vi "main(Test DQMH modules).bak.vi"() -> ()   [LabVIEW 2018, in "Application.lvlib"] (continued)
      tunnel: [w267 w1310 w1323 w1333 w1352 w1413 w1449 w1497 w1541 w1553 w1565 w1574 w1599 w1634 w1651 w1723 w1738 w1761 w1784 w1808 w1842 w1861 w1880 w1899 w1931 w1962 w1987 w2016 w2052 w2072 w2095 w2129 w2146 w2172 w2204 w2242 w2279 w2329 w2366 w2413 w2468 w2541 w2611 w2682 w2753 w2824 w2895 w2966 w3038 w3111 w3188 w3234 w3275 w3316 w3357 w3398 w3439 w3480 w3521 w3562 w3603 w3644 w3685 w3726 w3767 w3808 w3849 w3890 w3931 w3972 w4013 w4054 w4095 w4136 w4177 w4218 w4259 w4300 w4341 w4382 w4423 w4464 w4505 w4546 w4587 w4628 w4669 w4710 w4751 w4792 w4833 w4874 w4915 w4956 w4997 w5038 w5079 w5120 w5161 w5202 w5243 w5284 w5325 w5366 w5407 w5448 w5489 w5530 w5571 w5612 w5653 w5691 1 ("DUT channel (1-11)") 1 ("DUT channel (1-11)") 1 ("DUT channel (1-11)") 1 ("DUT channel (1-11)") 1 ("DUT channel (1-11)") 1 ("DUT channel (1-11)") 2 ("DUT channel (1-11)") 2 ("DUT channel (1-11)") 2 ("DUT channel (1-11)") 2 ("DUT channel (1-11)") 2 ("DUT channel (1-11)") 2 ("DUT channel (1-11)") 3 ("DUT channel (1-11)") 3 ("DUT channel (1-11)") 3 ("DUT channel (1-11)") 3 ("DUT channel (1-11)") 3 ("DUT channel (1-11)") 3 ("DUT channel (1-11)") 4 ("DUT channel (1-11)") 4 ("DUT channel (1-11)") 4 ("DUT channel (1-11)") 4 ("DUT channel (1-11)") 4 ("DUT channel (1-11)") 4 ("DUT channel (1-11)") 5 ("DUT channel (1-11)") 5 ("DUT channel (1-11)") 5 ("DUT channel (1-11)") 5 ("DUT channel (1-11)") 5 ("DUT channel (1-11)") 5 ("DUT channel (1-11)") 6 ("DUT channel (1-11)") 6 ("DUT channel (1-11)") 6 ("DUT channel (1-11)") 6 ("DUT channel (1-11)") 6 ("DUT channel (1-11)") 6 ("DUT channel (1-11)") 7 ("DUT channel (1-11)") 7 ("DUT channel (1-11)") 7 ("DUT channel (1-11)") 7 ("DUT channel (1-11)") 7 ("DUT channel (1-11)") 7 ("DUT channel (1-11)") 8 ("DUT channel (1-11)") 8 ("DUT channel (1-11)") 8 ("DUT channel (1-11)") 8 ("DUT channel (1-11)") 8 ("DUT channel (1-11)") 8 ("DUT channel (1-11)") 9 ("DUT channel (1-11)") 9 ("DUT channel (1-11)") 9 ("DUT channel (1-11)") 9 ("DUT channel (1-11)") 9 ("DUT channel (1-11)") 9 ("DUT channel (1-11)") 10 ("DUT channel (1-11)") 10 ("DUT channel (1-11)") 10 ("DUT channel (1-11)") 10 ("DUT channel (1-11)") 10 ("DUT channel (1-11)") 10 ("DUT channel (1-11)")] -> w236
      tunnel: w235 -> [w268 w1310 w1323 w1333 w1352 w1413 w1449 w1497 w1541 w1553 w1565 w1574 w1599 w1634 w1651 w1723 w1738 w1761 w1784 w1808 w1842 w1861 w1880 w1899 w1931 w1962 w1987 w2016 w2052 w2072 w2095 w2129 w2146 w2172 w2204 w2242 w2279 w2329 w2366 w2413 _ _ _ _ _ _ _ _ _ _ _ w3234 w3275 w3316 w3357 w3398 w3439 w3480 w3521 w3562 w3603 w3644 w3685 w3726 w3767 w3808 w3849 w3890 w3931 w3972 w4013 w4054 w4095 w4136 w4177 w4218 w4259 w4300 w4341 w4382 w4423 w4464 w4505 w4546 w4587 w4628 w4669 w4710 w4751 w4792 w4833 w4874 w4915 w4956 w4997 w5038 w5079 w5120 w5161 w5202 w5243 w5284 w5325 w5366 w5407 w5448 w5489 w5530 w5571 w5612 w5653 w5691 _ _ _ _ _ _ _ _ _ _ _ _ _ _ _ _ _ _ _ _ _ _ _ _ _ _ _ _ _ _ _ _ _ _ _ _ _ _ _ _ _ _ _ _ _ _ _ _ _ _ _ _ _ _ _ _ _ _ _ _]
      tunnel: [w265 w1309 w1322 w1332 w1354 w1401 w1448 w1496 w1540 w1552 w1564 w1573 w1598 w1633 w1650 w1722 w1737 w1760 w1783 w1807 w1841 w1860 w1879 w1898 w1930 w1961 w1986 w2015 w2051 w2071 w2094 w2128 w2145 w2171 w2207 w2241 w2278 w2328 w2357 w2412 w2446 w2540 w2610 w2681 w2752 w2823 w2894 w2965 w3037 w3110 w3187 w3229 w3271 w3312 w3353 w3394 w3438 w3476 w3517 w3558 w3599 w3640 w3681 w3722 w3763 w3804 w3845 w3885 w3929 w3968 w4009 w4050 w4091 w4132 w4173 w4214 w4255 w4296 w4337 w4378 w4418 w4460 w4501 w4542 w4583 w4624 w4665 w4706 w4747 w4787 w4829 w4870 w4911 w4952 w4993 w5033 w5075 w5115 w5157 w5197 w5238 w5280 w5321 w5361 w5403 w5444 w5485 w5526 w5567 w5608 w5649 w5690 w5698 w5755 w5812 w5868 w5926 w5982 w6039 w6096 w6153 w6210 w6267 w6324 w6382 w6439 w6496 w6553 w6610 w6667 w6724 w6781 w6837 w6895 w6951 w7008 w7066 w7122 w7180 w7236 w7294 w7350 w7407 w7464 w7522 w7579 w7635 w7692 w7749 w7806 w7863 w7920 w7977 w8034 w8091 w8151 w8205 w8263 w8319 w8377 w8434 w8491 w8547 w8604 w8661 w8718 w8775 w8832 w8893 w8952 w9011 w9070] -> w234
      tunnel: w233 -> [w266 w1309 w1322 w1332 w1354 w1401 w1448 w1496 w1540 w1552 w1564 w1573 w1598 w1633 w1650 w1722 w1737 w1760 w1783 w1807 w1841 w1860 w1879 w1898 w1930 w1961 w1986 w2015 w2051 w2071 w2094 w2128 w2145 w2171 w2207 w2241 w2278 w2328 w2357 w2412 w2446 w2540 w2610 w2681 w2752 w2823 w2894 w2965 w3037 w3110 w3187 _ _ _ _ _ _ _ _ _ _ _ _ _ _ _ _ _ _ _ _ _ _ _ _ _ _ _ _ _ _ _ _ _ _ _ _ _ _ _ _ _ _ _ _ _ _ _ _ _ _ _ _ _ _ _ _ _ _ _ _ w5690 _ _ _ _ _ _ _ _ _ _ _ _ _ _ _ _ _ _ _ _ _ _ _ _ _ _ _ _ _ _ _ _ _ _ _ _ _ _ _ _ _ _ _ _ _ _ _ _ _ _ _ _ _ _ _ _ _ _ _ _]
      tunnel: w230 -> [w273 _ _ _ _ _ _ _ _ _ _ _ _ _ _ _ _ _ _ _ _ _ _ _ _ _ _ _ w2043 _ _ _ _ _ _ _ _ _ _ _ _ _ _ _ _ _ _ _ _ _ _ _ _ _ _ _ _ _ _ _ _ _ _ _ _ _ _ _ _ _ _ _ _ _ _ _ _ _ _ _ _ _ _ _ _ _ _ _ _ _ _ _ _ _ _ _ _ _ _ _ _ _ _ _ _ _ _ _ _ _ _ _ _ _ _ _ _ _ _ _ _ _ _ _ _ _ _ _ _ _ _ _ _ _ _ _ _ _ _ _ _ _ _ _ _ _ _ _ _ _ _ _ _ _ _ _ _ _ _ _ _ _ _ _ _ _ _ _ _ _ _ _]
      tunnel: [_ _ _ _ _ _ _ _ _ _ _ _ _ _ _ _ _ _ _ _ _ _ _ _ _ _ _ _ _ _ _ _ _ _ _ _ _ _ TRUE _ _ _ _ _ _ _ _ _ _ _ _ _ _ _ _ _ _ _ _ _ _ _ _ _ _ _ _ _ _ _ _ _ _ _ _ _ _ _ _ _ _ _ _ _ _ _ _ _ _ _ _ _ _ _ _ _ _ _ _ _ _ _ _ _ _ _ _ _ _ _ _ _ _ _ _ _ _ _ _ _ _ _ _ _ _ _ _ _ _ _ _ _ _ _ _ _ _ _ _ _ _ _ _ _ _ _ _ _ _ _ _ _ _ _ _ _ _ _ _ _ _ _ _ _ _ _ _ _ _ _ _ _] -> w229
      tunnel: [w269 w1308 w1316 w1328 w1350 w1411 "Test Completed!!!!" w1488 w1539 w1551 w1563 w1571 w1594 w1632 "Initialize Apps" w1700 w1733 w1756 w1779 w1802 w1836 w1855 w1874 w1893 w1919 w1956 w1983 w2012 w2038 "HV-60D ready!!!!!!!!!!!!!!!!" w2088 w2125 w2140 w2164 w2201 w2236 w2271 w2321 w2359 "Shorted Circuit Test" "Test Channel 1" "Test Channel 2" "Test Channel 3" "Test Channel 4" "Test Channel 5" "Test Channel 6" "Test Channel 7" "Test Channel 8" "Test Channel 9" "Test Channel 10" "Test Channel 10" w3232 w3274 w3315 w3356 w3397 w3436 w3479 w3520 w3561 w3602 w3643 w3684 w3725 w3766 w3807 w3848 w3889 w3928 w3971 w4012 w4053 w4094 w4135 w4176 w4217 w4258 w4299 w4340 w4381 w4422 w4463 w4504 w4545 w4586 w4627 w4668 w4709 w4750 w4791 w4832 w4873 w4914 w4955 w4996 w5037 w5078 w5119 w5160 w5201 w5242 w5283 w5324 w5365 w5406 w5447 w5488 w5529 w5570 w5611 w5652 w5689 w5707 w5764 w5821 w5878 w5935 w5992 w6049 w6106 w6163 w6220 w6277 w6334 w6391 w6448 w6506 w6563 w6620 w6677 w6734 w6791 w6848 w6905 w6962 w7019 w7076 w7133 w7190 w7247 w7304 w7361 w7418 w7475 w7532 w7589 w7646 w7703 w7760 w7818 w7874 w7931 w7988 w8045 w8102 w8159 w8216 w8273 w8332 w8387 w8444 w8501 w8558 w8615 w8673 w8729 w8786 w8843 w8903 w8962 w9021 w9080] -> w226
      tunnel: w225 -> [w270 w1308 w1316 w1328 w1350 w1411 _ _ w1539 w1551 w1563 w1571 w1594 w1632 _ w1700 w1733 w1756 w1779 w1802 w1836 w1855 w1874 w1893 w1919 w1956 w1983 w2012 w2038 _ w2088 w2125 w2140 w2164 w2201 w2236 w2271 w2321 w2359 _ _ _ _ _ _ _ _ _ _ _ _ w3231 w3273 w3314 w3355 w3396 w3435 w3478 w3519 w3560 w3601 w3642 w3683 w3724 w3765 w3806 w3847 w3888 w3927 w3970 w4011 w4052 w4093 w4134 w4175 w4216 w4257 w4298 w4339 w4380 w4421 w4462 w4503 w4544 w4585 w4626 w4667 w4708 w4749 w4790 w4831 w4872 w4913 w4954 w4995 w5036 w5077 w5118 w5159 w5200 w5241 w5282 w5323 w5364 w5405 w5446 w5487 w5528 w5569 w5610 w5651 w5689 _ _ _ _ _ _ _ _ _ _ _ _ _ _ _ _ _ _ _ _ _ _ _ _ _ _ _ _ _ _ _ _ _ _ _ _ _ _ _ _ _ _ _ _ _ _ _ _ _ _ _ _ _ _ _ _ _ _ _ _]
      tunnel: w223 -> [_ _ _ _ _ _ w1427 _ _ _ _ _ _ _ _ _ _ _ _ _ _ _ _ _ _ _ _ _ _ _ _ _ _ _ _ _ _ _ _ _ _ _ _ _ _ _ _ _ _ _ _ _ _ _ _ _ _ _ _ _ _ _ _ _ _ _ _ _ _ _ _ _ _ _ _ _ _ _ _ _ _ _ _ _ _ _ _ _ _ _ _ _ _ _ _ _ _ _ _ _ _ _ _ _ _ _ _ _ _ _ _ _ _ _ _ _ _ _ _ _ _ _ _ _ _ _ _ _ _ _ _ _ _ _ _ _ _ _ _ _ _ _ _ _ _ _ _ _ _ _ _ _ _ _ _ _ _ _ _ _ _ _ _ _ _ _ _ _ _ _ _ _]
      frame "Apps.WaitForEvent", Default {
        n141 = event shown="[26] <CE14_v2 Broadcast Events.CE14 response data>: User Event" {
          selector: w282 -> [_ w310 _ _ _ _ _ _ _ _ _ _ _ _ _ _ _ _ _ _ _ _ _ _ _ _ _ _ _ _ _ _ _ _ _ _ _ _ _ _ _ _]
          dyn-events: [_ w310 _ _ _ _ _ _ _ _ _ _ _ _ _ _ _ _ _ _ _ _ _ _ _ _ _ _ _ _ _ _ _ _ _ _ _ _ _ _ _ _] -> w281
          timeout: w271 -> [_ _ _ _ _ _ _ _ _ _ _ _ _ _ _ _ _ _ _ _ _ _ _ _ _ _ _ _ _ _ _ _ _ _ _ _ _ _ _ _ _ _]
          tunnel: [w289 w305 w323 w346 w361 w379 w394 w479 w491 w502 w510 w532 w551 w568 w580 w601 w623 w658 w677 w694 w718 w737 w756 w785 w825 w845 w873 w981 w1012 w1035 w1056 w1077 w1098 w1119 w1140 w1161 w1182 w1203 w1224 w1240 w1265 w1290] -> w283
          tunnel: w271 -> [w289 w305 w324 w346 w361 w379 w393 w479 w491 w502 w510 w532 w551 w568 w580 w601 w623 w658 w677 w694 w718 w737 w756 w785 w825 w845 w873 w981 w1012 w1035 w1056 w1077 w1098 w1119 w1140 w1161 w1182 w1203 w1224 w1240 w1265 w1290]
          tunnel: [w293 w309 _ w337 _ w376 w384 w473 w483 w497 w508 w527 w546 w560 w576 w599 w621 w651 w672 w691 w716 w735 w754 w779 w817 w839 w869 w980 w1009 w1033 w1054 w1075 w1096 w1117 w1138 w1159 w1180 w1201 w1222 w1238 w1262 w1287] -> w279
          tunnel: w278 -> [w287 w309 _ w339 _ w378 w398 w474 w485 w501 w507 w526 w545 w561 w575 w598 w620 w650 w671 w690 w715 w734 w753 w778 w819 w843 w868 w979 w1010 w1034 w1055 w1076 w1097 w1118 w1139 w1160 w1181 w1202 w1223 w1237 w1261 w1288]
          tunnel: w277 -> [w290 w303 w325 w341 _ w367 w400 w477 w487 w500 w513 w531 w550 _ w570 w606 w627 w655 w676 w702 w721 w740 w761 w782 w824 w846 w870 w969 w1006 w1030 w1051 w1072 w1093 w1114 w1135 w1157 w1177 w1198 w1219 w1231 w1256 w1281]
          tunnel: [w294 w312 w330 w345 w360 w375 w399 w478 w489 w495 w509 w529 w547 w567 w577 w600 w622 w652 w673 w693 w717 w736 w755 w784 w820 w840 w871 w982 w1005 w1028 w1049 w1070 w1091 w1112 w1133 w1155 w1175 w1196 w1217 w1239 w1264 w1289] -> w276
          tunnel: w275 -> [w294 w312 w330 w345 w360 w375 w399 w478 w489 w495 w509 w529 w547 w567 w577 w600 w622 w652 w673 w693 w717 w736 w755 w784 w820 _ w872 w982 w1005 w1028 w1049 w1070 w1091 w1112 w1133 w1155 w1175 w1196 w1217 w1239 w1264 w1289]
          tunnel: w274 -> [_ _ _ w335 _ _ w386 _ _ _ _ _ _ _ _ _ _ _ _ _ _ _ _ _ _ _ _ _ _ w1027 w1046 w1066 w1087 w1108 w1129 w1150 w1171 w1192 w1213 _ _ _]
          tunnel: w272 -> [w292 w311 _ _ _ _ _ _ _ _ w506 w525 w544 _ w574 w597 w619 w649 w670 w689 w714 w733 w752 w777 w816 w841 w866 w978 _ _ _ _ _ _ _ _ _ _ _ w1236 w1263 w1286]
          tunnel: w273 -> [_ _ _ _ _ _ _ _ _ _ _ _ _ _ _ _ _ _ _ _ _ _ _ _ _ _ _ _ _ _ _ _ _ _ _ _ _ _ _ _ _ _]
          tunnel: w268 -> [w285 w307 w328 w343 w358 w373 w388 w471 w481 w493 w504 w523 w542 w565 w572 w595 _ w647 w668 w687 w712 w731 w750 w774 w814 w835 w863 w965 w1003 _ _ _ _ _ _ _ _ _ _ w1234 w1259 w1284]
          tunnel: w270 -> [w286 _ w329 w344 w359 w374 _ _ w482 w494 w505 w524 w543 w566 w573 w596 w618 w648 w669 w688 w713 w732 w751 w776 w815 w836 w864 w966 w1004 w1023 w1044 w1065 w1086 w1107 w1128 w1149 w1170 w1191 w1212 w1235 w1260 w1285]
          tunnel: [w286 "Wait for JIG lock" w329 w344 w359 w374 "Start Auto Test" "Settings" w482 w494 w505 w524 w543 w566 w573 w596 w618 w648 w669 w688 w713 w732 w751 w776 w815 w836 w864 w966 w1004 w1023 w1044 w1065 w1086 w1107 w1128 w1149 w1170 w1191 w1212 w1235 w1260 w1285] -> w269
          tunnel: [w285 w307 w328 w343 w358 w373 w388 w471 w481 w493 w504 w523 w542 w565 w572 w595 w615 w647 w668 w687 w712 w731 w750 w774 w814 w835 w862 w965 w1003 1 ("DUT channel (1-11)") 2 ("DUT channel (1-11)") 3 ("DUT channel (1-11)") 4 ("DUT channel (1-11)") 5 ("DUT channel (1-11)") 6 ("DUT channel (1-11)") 7 ("DUT channel (1-11)") 8 ("DUT channel (1-11)") 9 ("DUT channel (1-11)") 10 ("DUT channel (1-11)") w1234 w1259 w1284] -> w267
          tunnel: w266 -> [w284 w306 w327 w342 w357 w372 w387 w470 w480 w492 w503 w522 w541 w564 w571 w594 w617 w646 w667 w686 w711 w730 w749 _ w813 w834 w858 w964 w1002 w1021 w1042 w1063 w1084 w1105 w1126 w1147 w1168 w1189 w1210 w1230 w1255 w1280]
          tunnel: [w284 w306 w327 w342 w357 w372 w387 w470 w480 w492 w503 w522 w541 w564 w571 w594 w617 w646 w667 w686 w711 w730 w749 w770 w813 w834 w857 w964 w1002 w1021 w1042 w1063 w1084 w1105 w1126 w1147 w1168 w1189 w1210 w1230 w1255 w1280] -> w265
          tunnel: w264 -> [_ _ _ _ _ _ _ _ _ _ _ _ _ _ _ _ _ _ _ _ _ _ _ _ _ _ w861 _ _ _ _ _ _ _ _ _ _ _ _ _ _ _]
          event Timeout {
            n142 = event-data() -> ()  [unwired: 1 in, 1 out]
            n143 = disable-structure shown="LOGGING==TRUE" {
              disable-tunnel: w292 -> [w295 _]
              frame condition #0 (active) {
                n144 = Empty String/Path?(string/path=w295) -> (empty?=w302:bool)
                n145 = Select(t="Quece timeout", s=w302, f=w295) -> (s? t:f=w300:string)
                n146 = Format Into String(format string=": %s", initial string=w300, "UI timeout") -> (resulting string=w297:string)  [unwired: 1 in, 1 out]
                n147 = call "string log (SubVI).vi"("Enum"=enum16{"Init", "Log", "Read"}."Log", "state Name"=w297) -> ()  [unwired: 8 in, 2 out]
              }
              frame condition #1 {
              }
            }
            n148 = call "App enquece.vi"("command"="Apps.WaitingForTrigger", "queue in"=w290) -> ("error out"=w288:errorcluster)  [unwired: 8 in, 1 out]
            n149 = Merge Errors(w287, w288) -> (w293:errorcluster)
          }
          event "Test": Value Change {
            n150 = event-data() -> ()  [unwired: 1 in, 2 out]
            n151 = disable-structure shown="Default" {
              disable-tunnel: w311 -> [w315 _]
              frame condition #0 (active) {
                n152 = Empty String/Path?(string/path=w315) -> (empty?=w322:bool)
                n153 = Select(t="Quece timeout", s=w322, f=w315) -> (s? t:f=w320:string)
                n154 = Format Into String(format string=": %s", initial string=w320, "Test") -> (resulting string=w317:string)  [unwired: 1 in, 1 out]
                n155 = call "string log (SubVI).vi"("Enum"=enum16{"Init", "Log", "Read"}."Log", "state Name"=w317) -> ()  [unwired: 8 in, 2 out]
              }
              frame condition #1 {
              }
            }
            n156 = call "App enquece.vi"("command"="Apps.AutoMode", "queue in"=w303) -> ()  [unwired: 8 in, 2 out]
            n157 = disable-structure shown="Disabled" {
              frame Disabled {
                n158 = Select(t=100, f=-1) -> ()  [unwired: 1 in, 1 out]
              }
              frame Enabled {
              }
            }
          }
          event "Auto/Man": Value Change {
            n159 = event-data() -> ("NewVal"=w326:bool)  [unwired: 1 in, 5 out]
            n160 = case shown="True" w326 {
              tunnel: w325 -> [_ w333]
              tunnel: [-1 w332] -> w323
              tunnel: w324 -> [_ w332]
              frame False {
              }
              frame True {
                n161 = call "App enquece.vi"("command"="Apps.AutoMode", "queue in"=w333) -> ()  [unwired: 8 in, 2 out]
              }
            }
          }
          event "Test Single DRV": Value Change {
            n162 = event-data() -> ()  [unwired: 1 in, 1 out]
            n163 = case shown="1.." "DRV number" {
              selector: "DRV number" -> [_ w349]
              tunnel: ["MEAS.AllRelaysOFF" w352] -> w340
              tunnel: w335 -> [w347 _]
              frame 0, Default {
                n164 = call "reset DRV UI (SubVI).vi"("Ref  in"=w347) -> ()  [unwired: 9 in, 2 out]
              }
              frame 1.. {
                n165 = Format Into String(format string="%d%s", initial string="Test DRV ", w349, "A" ("input 3")) -> (resulting string=w352:string)  [unwired: 1 in, 1 out]
              }
            }
            n166 = call "App enquece.vi"("command"=w340, "queue in"=w341) -> ("error out"=w338:errorcluster)  [unwired: 8 in, 1 out]
            n167 = Merge Errors(w339, w338) -> (w337:errorcluster)
          }
          event "DMM query": Value Change {
            n168 = event-data() -> ()  [unwired: 1 in, 6 out]
            n169 = flat-sequence {
              tunnel: [w364] -> w355
              frame #0 {
                w362 = ""
                n170 = Wait (ms)(milliseconds to wait=u32 100) -> ()  [unwired: 1 out]
                n171 = local write "DMM func?"(w362) -> ()
                n172 = local write "DMM range?"(w362) -> ()
                n173 = xnode "Error Ring"() -> ("error out"=w364:errorcluster)
              }
            }
            n174 = call "Query func.vi"("error in"=w355) -> ("String"=→"DMM func?":string)  [unwired: 8 in, 2 out]
            n175 = call "query range.vi"("error in"=w355) -> ("String"=→"DMM range?":string)  [unwired: 8 in, 2 out]
          }
          event "VIEW": Value Change {
            n176 = event-data() -> ()  [unwired: 1 in, 1 out]
            n177 = disable-structure shown="Disabled" {
              frame Disabled {
                n178 = Initialize Array(FALSE, 6 ("dimension size"), 10 ("dimension size")) -> (w380:bool[][])
                n179 = local write "Short DRV"(w380) -> ()
              }
              frame Enabled {
              }
            }
            n180 = call "App enquece.vi"("command"="Apps.UI Update 1", "queue in"=w367) -> ()  [unwired: 8 in, 2 out]
            n181 = invoke class="VI" method="FP.Open"("State"=T18."Hidden") -> (error out=w371:errorcluster)  [unwired: 4 in, 4 out]
            n182 = call "View DRV data.vi"("error in (no error)"=w371) -> ("error out"=w370:errorcluster)  [unwired: 10 in]
            n183 = invoke class="VI" method="FP.Open"(error in=w370, "State"=T18."Standard") -> (error out=w377:errorcluster)  [unwired: 3 in, 4 out]
            n184 = Merge Errors(w378, w377) -> (w376:errorcluster)
          }
          event User Event {
            # "#HungNotes:\nStart HV60D from this frame (check new board  installed)"
            # "Stop Timeout event"
            n185 = event-data() -> ("new board?"=w392:bool, "new trigger"=→"new Trigger?":bool, "last trigger"=→"last Trigger?":bool)  [unwired: 1 in, 1 out]
            "New board?" <- w392
            n186 = call "reset DRV UI (SubVI).vi"("Ref  in"=w386) -> ()  [unwired: 9 in, 2 out]
            n187 = case shown="True" w392 {
              tunnel: w400 -> [_ w402]
              tunnel: [_ w401] -> w385
              frame False {
              }
              frame True {
                n188 = case shown="\"Pinpoint_JIG\"" "Enum" {
                  tunnel: [w416 w433 w444 w463] -> w403
                  frame "All DRV" {
                    n189 = Build Array("Test Shorted Circuits", "Timer Start", "Test Channel 1", "Test Channel 2", "Test Channel 3", "Test Channel 4", "Test Channel 5", "Test Channel 6") -> (w408:string[])
                    n190 = Build Array("Test Channel 7", "Test Channel 8", "Test Channel 9", "Test Channel 10", "Timer Stop") -> (w417:string[])
                    n191 = Build Array("MEAS.AllRelaysOFF", "MEAS.Reset JIG", "Apps.UI Update 2") -> (w409:string[])
                    n192 = Build Array (concatenate)(w408, w417, w409) -> (w416:string[])
                  }
                  frame "Fixxed" {
                    n193 = Build Array("Test Shorted Circuits", "Timer Start", "Test Channel 1", "Test Channel 2", "Test Channel 3", "Test Channel 4", "Test Channel 5", "Test Channel 6", "Test Channel 7") -> (w435:string[])
                    n194 = Build Array("MEAS.AllRelaysOFF", "MEAS.Reset JIG", "Apps.UI Update 2") -> (w429:string[])
                    n195 = Build Array (concatenate)(w435, "Timer Stop", w429) -> (w433:string[])
                  }
                  frame "Pinpoint_JIG" {
                    n196 = Build Array("Test Channel 8", "Test Channel 9", "Test Channel 10") -> (w448:string[])
                    n197 = Build Array("Test Shorted Circuits", "Timer Start") -> (w445:string[])
                    n198 = Build Array("MEAS.AllRelaysOFF", "MEAS.Reset JIG", "Apps.UI Update 2") -> (w447:string[])
                    n199 = Build Array (concatenate)(w445, w448, "Timer Stop", w447) -> (w444:string[])
                  }
                  frame "00037845(M26)" {
                    n200 = Build Array("Test Channel 8", "Test Channel 9", "Test Channel 10A", "Timer Stop") -> (w458:string[])
                    n201 = Build Array("Test Shorted Circuits", "Timer Start") -> (w464:string[])
                    n202 = Build Array("MEAS.AllRelaysOFF", "MEAS.Reset JIG", "Apps.UI Update 2") -> (w457:string[])
                    n203 = Build Array (concatenate)(w464, w458, w457) -> (w463:string[])
                  }
                }
                n204 = for {
                  tunnel: [w407] -> w401 mode=indexing
                  tunnel: w403 -> [w406] mode=indexing
                  tunnel: w402 -> [w405]
                  n205 = call "App enquece.vi"("command"=w406, "queue in"=w405) -> ("error out"=w407:errorcluster)  [unwired: 8 in, 1 out]
                }
              }
            }
            n206 = control-ref of="DRV 61"() -> (w390:refnum<vi>)
            n207 = property class="ColBox"(reference=w390, "Value"=u32 10000536 ("DRV 1")) -> ()  [unwired: 1 in, 2 out]
            n208 = Select(t=-1, s=w392, f=w393) -> (s? t:f=w394:i32)
            n209 = Merge Errors(w398, w385) -> (w384:errorcluster)
          }
          event "Settings": Value Change {
            n210 = event-data() -> ()  [unwired: 1 in, 6 out]
            n211 = call "App enquece.vi"("command"="INIT.Read DRV code", "queue in"=w477) -> ("error out"=w475:errorcluster)  [unwired: 8 in, 1 out]
            n212 = Merge Errors(w474, w475) -> (w473:errorcluster)
          }
          event Panel Close? {
            n213 = event-data() -> ()  [unwired: 1 in, 4 out]
            n214 = call "App enquece.vi"("Priority Enquece"=TRUE, "command"="Apps.Exit", "queue in"=w487) -> ("error out"=w484:errorcluster)  [unwired: 7 in, 1 out]
            n215 = Merge Errors(w485, w484) -> (w483:errorcluster)
            n216 = event-data("Discard?"=TRUE) -> ()  [unwired: 1 in, 1 out]
          }
          event "Exit": Value Change {
            n217 = event-data() -> ()  [unwired: 1 in, 1 out]
            n218 = call "App enquece.vi"("Priority Enquece"=TRUE, "command"="Apps.Exit", "queue in"=w500) -> ("error out"=w499:errorcluster)  [unwired: 7 in, 1 out]
            n219 = Merge Errors(w501, w499) -> (w497:errorcluster)
          }
          event "check connected": Value Change {
            n220 = event-data() -> ()  [unwired: 1 in, 1 out]
            n221 = disable-structure shown="LOGGING==TRUE" {
              disable-tunnel: w506 -> [w514 _]
              frame condition #0 (active) {
                n222 = Empty String/Path?(string/path=w514) -> (empty?=w521:bool)
                n223 = Select(t="Quece timeout", s=w521, f=w514) -> (s? t:f=w519:string)
                n224 = Format Into String(format string=": %s", initial string=w519, "Check connected") -> (resulting string=w516:string)  [unwired: 1 in, 1 out]
                n225 = call "string log (SubVI).vi"("Enum"=enum16{"Init", "Log", "Read"}."Log", "state Name"=w516) -> ()  [unwired: 8 in, 2 out]
              }
              frame condition #1 {
              }
            }
            n226 = call "App enquece.vi"("command"="MEAS.Read EMIC connected", "queue in"=w513) -> ("error out"=w511:errorcluster)  [unwired: 8 in, 1 out]
            n227 = Merge Errors(w507, w511) -> (w508:errorcluster)
          }
          event "Open COM eMIC": Value Change {
            n228 = event-data() -> ()  [unwired: 1 in, 1 out]
            n229 = disable-structure shown="LOGGING==TRUE" {
              disable-tunnel: w525 -> [w533 _]
              frame condition #0 (active) {
                n230 = Empty String/Path?(string/path=w533) -> (empty?=w540:bool)
                n231 = Select(t="Quece timeout", s=w540, f=w533) -> (s? t:f=w538:string)
                n232 = Format Into String(format string=": %s", initial string=w538, "Open COM eMIC") -> (resulting string=w535:string)  [unwired: 1 in, 1 out]
                n233 = call "string log (SubVI).vi"("Enum"=enum16{"Init", "Log", "Read"}."Log", "state Name"=w535) -> ()  [unwired: 8 in, 2 out]
              }
              frame condition #1 {
              }
            }
            n234 = call "App enquece.vi"("command"="INIT.Open COM EMIC", "queue in"=w531) -> ("error out"=w530:errorcluster)  [unwired: 8 in, 1 out]
            n235 = Merge Errors(w526, w530) -> (w527:errorcluster)
          }
          event "Read trigger": Value Change {
            n236 = event-data() -> ()  [unwired: 1 in, 1 out]
            n237 = disable-structure shown="LOGGING==TRUE" {
              disable-tunnel: w544 -> [w552 _]
              frame condition #0 (active) {
                n238 = Empty String/Path?(string/path=w552) -> (empty?=w559:bool)
                n239 = Select(t="Quece timeout", s=w559, f=w552) -> (s? t:f=w557:string)
                n240 = Format Into String(format string=": %s", initial string=w557, "Read Trigger") -> (resulting string=w554:string)  [unwired: 1 in, 1 out]
                n241 = call "string log (SubVI).vi"("Enum"=enum16{"Init", "Log", "Read"}."Log", "state Name"=w554) -> ()  [unwired: 8 in, 2 out]
              }
              frame condition #1 {
              }
            }
            n242 = call "App enquece.vi"("command"="MEAS.Read TRIGGER", "queue in"=w550) -> ("error out"=w548:errorcluster)  [unwired: 8 in, 1 out]
            n243 = Merge Errors(w545, w548) -> (w546:errorcluster)
          }
          event "Set trigger value": Value Change {
            n244 = event-data() -> ()  [unwired: 1 in, 6 out]
            n245 = call "SET trigger value.vi"("Boolean"="set value") -> ("error out"=w562:errorcluster)  [unwired: 10 in]
            n246 = Merge Errors(w561, w562) -> (w560:errorcluster)
          }
          event "Read Optos": Value Change {
            n247 = event-data() -> ()  [unwired: 1 in, 1 out]
            n248 = disable-structure shown="LOGGING==TRUE" {
              disable-tunnel: w574 -> [w586 _]
              frame condition #0 (active) {
                n249 = Empty String/Path?(string/path=w586) -> (empty?=w593:bool)
                n250 = Select(t="Quece timeout", s=w593, f=w586) -> (s? t:f=w591:string)
                n251 = Format Into String(format string=": %s", initial string=w591, "Read Optos") -> (resulting string=w588:string)  [unwired: 1 in, 1 out]
                n252 = call "string log (SubVI).vi"("Enum"=enum16{"Init", "Log", "Read"}."Log", "state Name"=w588) -> ()  [unwired: 8 in, 2 out]
              }
              frame condition #1 {
              }
            }
            n253 = flat-sequence {
              tunnel: w570 -> [w581]
              tunnel: [w581] -> w569
              frame #0 {
                n254 = Initialize Array(FALSE, 6 ("dimension size"), 10 ("dimension size")) -> (w585:bool[][])
                n255 = local write "Short DRV"(w585) -> ()
              }
            }
            n256 = call "App enquece.vi"("command"="MEAS.Read Optos", "queue in"=w569) -> ("error out"=w578:errorcluster)  [unwired: 8 in, 1 out]
            n257 = Merge Errors(w575, w578) -> (w576:errorcluster)
          }
          event "Select DMM's Current Input": Value Change {
            n258 = event-data() -> ()  [unwired: 1 in, 1 out]
            n259 = disable-structure shown="LOGGING==TRUE" {
              disable-tunnel: w597 -> [w607 _]
              frame condition #0 (active) {
                n260 = Empty String/Path?(string/path=w607) -> (empty?=w614:bool)
                n261 = Select(t="Quece timeout", s=w614, f=w607) -> (s? t:f=w612:string)
                n262 = Format Into String(format string=": %s", initial string=w612, "DMM Current Input") -> (resulting string=w609:string)  [unwired: 1 in, 1 out]
                n263 = call "string log (SubVI).vi"("Enum"=enum16{"Init", "Log", "Read"}."Log", "state Name"=w609) -> ()  [unwired: 8 in, 2 out]
              }
              frame condition #1 {
              }
            }
            n264 = To Variant(anything="mux2-1(DMM I) encode") -> (Variant=w603:variant)
            n265 = call "App enquece.vi"("command data"=w603, "command"="MEAS.Sel Input Current", "queue in"=w606) -> ("error out"=w602:errorcluster)  [unwired: 7 in, 1 out]
            n266 = Merge Errors(w598, w602) -> (w599:errorcluster)
          }
          event "DEMUX 1-10": Value Change {
            n267 = event-data() -> ()  [unwired: 1 in, 1 out]
            n268 = disable-structure shown="LOGGING==TRUE" {
              disable-tunnel: w619 -> [w638 _]
              frame condition #0 (active) {
                n269 = Empty String/Path?(string/path=w638) -> (empty?=w645:bool)
                n270 = Select(t="Quece timeout", s=w645, f=w638) -> (s? t:f=w643:string)
                n271 = Format Into String(format string=": %s", initial string=w643, "demux1-10") -> (resulting string=w640:string)  [unwired: 1 in, 1 out]
                n272 = call "string log (SubVI).vi"("Enum"=enum16{"Init", "Log", "Read"}."Log", "state Name"=w640) -> ()  [unwired: 8 in, 2 out]
              }
              frame condition #1 {
              }
            }
            n273 = To Variant(anything="demux1_10(x6)_encode") -> (Variant=w625:variant)
            n274 = case shown="\"demux1_10_channel0\", Default" "demux1_10(x6)_encode" {
              tunnel: [_ 1 ("DUT channel (1-11)") 2 ("DUT channel (1-11)") 3 ("DUT channel (1-11)") 4 ("DUT channel (1-11)") 5 ("DUT channel (1-11)") 6 ("DUT channel (1-11)") 7 ("DUT channel (1-11)") 8 ("DUT channel (1-11)") 9 ("DUT channel (1-11)") 10 ("DUT channel (1-11)")] -> w615
              frame "demux1_10_channel0", Default {
              }
              frame "demux1_10_channel1" {
              }
              frame "demux1_10_channel2" {
              }
              frame "demux1_10_channel3" {
              }
              frame "demux1_10_channel4" {
              }
              frame "demux1_10_channel5" {
              }
              frame "demux1_10_channel6" {
              }
              frame "demux1_10_channel7" {
              }
              frame "demux1_10_channel8" {
              }
              frame "demux1_10_channel9" {
              }
              frame "demux1_10_channel10" {
              }
            }
            n275 = call "App enquece.vi"("command data"=w625, "command"="MEAS.demux1-10", "queue in"=w627) -> ("error out"=w624:errorcluster)  [unwired: 7 in, 1 out]
            n276 = Merge Errors(w620, w624) -> (w621:errorcluster)
          }
          event "eMIC": Value Change {
            n277 = event-data() -> ()  [unwired: 1 in, 1 out]
            n278 = disable-structure shown="LOGGING==TRUE" {
              disable-tunnel: w649 -> [w659 _]
              frame condition #0 (active) {
                n279 = Empty String/Path?(string/path=w659) -> (empty?=w666:bool)
                n280 = Select(t="Quece timeout", s=w666, f=w659) -> (s? t:f=w664:string)
                n281 = Format Into String(format string=": %s", initial string=w664, "eMIC") -> (resulting string=w661:string)  [unwired: 1 in, 1 out]
                n282 = call "string log (SubVI).vi"("Enum"=enum16{"Init", "Log", "Read"}."Log", "state Name"=w661) -> ()  [unwired: 8 in, 2 out]
              }
              frame condition #1 {
              }
            }
            n283 = To Variant(anything="eMIC 6 values") -> (Variant=w653:variant)
            n284 = call "App enquece.vi"("command data"=w653, "command"="MEAS.eMIC", "queue in"=w655) -> ("error out"=w657:errorcluster)  [unwired: 7 in, 1 out]
            n285 = Merge Errors(w650, w657) -> (w651:errorcluster)
          }
          event "connect DMM": Value Change {
            n286 = event-data() -> ()  [unwired: 1 in, 1 out]
            n287 = disable-structure shown="LOGGING==TRUE" {
              disable-tunnel: w670 -> [w678 _]
              frame condition #0 (active) {
                n288 = Empty String/Path?(string/path=w678) -> (empty?=w685:bool)
                n289 = Select(t="Quece timeout", s=w685, f=w678) -> (s? t:f=w683:string)
                n290 = Format Into String(format string=": %s", initial string=w683, "Connect DMM") -> (resulting string=w680:string)  [unwired: 1 in, 1 out]
                n291 = call "string log (SubVI).vi"("Enum"=enum16{"Init", "Log", "Read"}."Log", "state Name"=w680) -> ()  [unwired: 8 in, 2 out]
              }
              frame condition #1 {
              }
            }
            n292 = call "App enquece.vi"("command"="INIT.Open COM DMM", "queue in"=w676) -> ("error out"=w675:errorcluster)  [unwired: 8 in, 1 out]
            n293 = Merge Errors(w671, w675) -> (w672:errorcluster)
          }
          event "config DMM": Value Change {
            n294 = event-data() -> ()  [unwired: 1 in, 1 out]
            n295 = disable-structure shown="LOGGING==TRUE" {
              disable-tunnel: w689 -> [w703 _]
              frame condition #0 (active) {
                n296 = Empty String/Path?(string/path=w703) -> (empty?=w710:bool)
                n297 = Select(t="Quece timeout", s=w710, f=w703) -> (s? t:f=w708:string)
                n298 = Format Into String(format string=": %s", initial string=w708, "config DMM") -> (resulting string=w705:string)  [unwired: 1 in, 1 out]
                n299 = call "string log (SubVI).vi"("Enum"=enum16{"Init", "Log", "Read"}."Log", "state Name"=w705) -> ()  [unwired: 8 in, 2 out]
              }
              frame condition #1 {
              }
            }
            n300 = Bundle By Name(cluster=T19 {"DMM config cluster"={"DCV range"=0.0, "DCI range"=0.0, "Detector Rate"=0}, "mux2-1(DMM I) encode"=enum."DMM I (0.5)"} ("DMM all config"), "DMM config cluster.DCV range"="DCV range", "DMM config cluster.DCI range"="DCI range", "DMM config cluster.Detector Rate"="Detector Rate") -> (w697:T19)
            n301 = To Variant(anything=w697) -> (Variant=w695:variant)
            n302 = call "App enquece.vi"("command data"=w695, "command"="MEAS.Set DMM config", "queue in"=w702) -> ("error out"=w692:errorcluster)  [unwired: 7 in, 1 out]
            n303 = Merge Errors(w690, w692) -> (w691:errorcluster)
          }
          event "DMM read dual value": Value Change {
            n304 = event-data() -> ()  [unwired: 1 in, 1 out]
            n305 = disable-structure shown="LOGGING==TRUE" {
              disable-tunnel: w714 -> [w722 _]
              frame condition #0 (active) {
                n306 = Empty String/Path?(string/path=w722) -> (empty?=w729:bool)
                n307 = Select(t="Quece timeout", s=w729, f=w722) -> (s? t:f=w727:string)
                n308 = Format Into String(format string=": %s", initial string=w727, "DMM read dual value") -> (resulting string=w724:string)  [unwired: 1 in, 1 out]
                n309 = call "string log (SubVI).vi"("Enum"=enum16{"Init", "Log", "Read"}."Log", "state Name"=w724) -> ()  [unwired: 8 in, 2 out]
              }
              frame condition #1 {
              }
            }
            n310 = call "App enquece.vi"("command"="MEAS.DMM dual read", "queue in"=w721) -> ("error out"=w719:errorcluster)  [unwired: 8 in, 1 out]
            n311 = Merge Errors(w715, w719) -> (w716:errorcluster)
          }
          event "Reset JIG": Value Change {
            n312 = event-data() -> ()  [unwired: 1 in, 1 out]
            n313 = disable-structure shown="LOGGING==TRUE" {
              disable-tunnel: w733 -> [w741 _]
              frame condition #0 (active) {
                n314 = Empty String/Path?(string/path=w741) -> (empty?=w748:bool)
                n315 = Select(t="Quece timeout", s=w748, f=w741) -> (s? t:f=w746:string)
                n316 = Format Into String(format string=": %s", initial string=w746, "reset JIG") -> (resulting string=w743:string)  [unwired: 1 in, 1 out]
                n317 = call "string log (SubVI).vi"("Enum"=enum16{"Init", "Log", "Read"}."Log", "state Name"=w743) -> ()  [unwired: 8 in, 2 out]
              }
              frame condition #1 {
              }
            }
            n318 = call "App enquece.vi"("command"="MEAS.Reset JIG", "queue in"=w740) -> ("error out"=w738:errorcluster)  [unwired: 8 in, 1 out]
            n319 = Merge Errors(w734, w738) -> (w735:errorcluster)
          }
          event "TurnON/OFF +5V": Value Change {
            n320 = event-data() -> ()  [unwired: 1 in, 1 out]
            n321 = disable-structure shown="LOGGING==TRUE" {
              disable-tunnel: w752 -> [w762 _]
              frame condition #0 (active) {
                n322 = Empty String/Path?(string/path=w762) -> (empty?=w769:bool)
                n323 = Select(t="Quece timeout", s=w769, f=w762) -> (s? t:f=w767:string)
                n324 = Format Into String(format string=": %s", initial string=w767, "ON/OFF +5V") -> (resulting string=w764:string)  [unwired: 1 in, 1 out]
                n325 = call "string log (SubVI).vi"("Enum"=enum16{"Init", "Log", "Read"}."Log", "state Name"=w764) -> ()  [unwired: 8 in, 2 out]
              }
              frame condition #1 {
              }
            }
            n326 = To Variant(anything="5V Value") -> (Variant=w758:variant)
            n327 = call "App enquece.vi"("command data"=w758, "command"="MEAS.Turn+5V", "queue in"=w761) -> ("error out"=w760:errorcluster)  [unwired: 7 in, 1 out]
            n328 = Merge Errors(w753, w760) -> (w754:errorcluster)
          }
          event "mux 6-1": Value Change {
            n329 = event-data() -> ()  [unwired: 1 in, 1 out]
            n330 = disable-structure shown="LOGGING==TRUE" {
              disable-tunnel: w777 -> [w805 _]
              frame condition #0 (active) {
                n331 = Empty String/Path?(string/path=w805) -> (empty?=w812:bool)
                n332 = Select(t="Quece timeout", s=w812, f=w805) -> (s? t:f=w810:string)
                n333 = Format Into String(format string=": %s", initial string=w810, "mux6-1") -> (resulting string=w807:string)  [unwired: 1 in, 1 out]
                n334 = call "string log (SubVI).vi"("Enum"=enum16{"Init", "Log", "Read"}."Log", "state Name"=w807) -> ()  [unwired: 8 in, 2 out]
              }
              frame condition #1 {
              }
            }
            n335 = Decrement(x=w774) -> (x-1=w773:i32)
            n336 = Multiply(x=w773, y=6) -> (x*y=w771:i32)
            n337 = case shown="\"mux6_1_channel6_3\"" "mux 6-1 data" {
              tunnel: w771 -> [_ w789 w792 w795 w798 w801 w804]
              tunnel: [0 w787 w790 w793 w796 w799 w802] -> w770
              frame "mux6-1_channel0", Default {
              }
              frame "mux6_1_channel1_3" {
                n338 = Add(x=w789, y=0) -> (x+y=w787:i32)
              }
              frame "mux6_1_channel2_3" {
                n339 = Add(x=w792, y=1) -> (x+y=w790:i32)
              }
              frame "mux6_1_channel3_3" {
                n340 = Add(x=w795, y=2) -> (x+y=w793:i32)
              }
              frame "mux6_1_channel4_3" {
                n341 = Add(x=w798, y=3) -> (x+y=w796:i32)
              }
              frame "mux6_1_channel5_3" {
                n342 = Add(x=w801, y=4) -> (x+y=w799:i32)
              }
              frame "mux6_1_channel6_3" {
                n343 = Add(x=w804, y=5) -> (x+y=w802:i32)
              }
            }
            n344 = To Variant(anything="mux 6-1 data") -> (Variant=w781:variant)
            n345 = call "App enquece.vi"("command data"=w781, "command"="MEAS.mux6_1", "queue in"=w782) -> ("error out"=w780:errorcluster)  [unwired: 7 in, 1 out]
            n346 = Merge Errors(w778, w780) -> (w779:errorcluster)
          }
          event "Mux 10-1": Value Change {
            n347 = event-data() -> ()  [unwired: 1 in, 1 out]
            n348 = disable-structure shown="LOGGING==TRUE" {
              disable-tunnel: w816 -> [w826 _]
              frame condition #0 (active) {
                n349 = Empty String/Path?(string/path=w826) -> (empty?=w833:bool)
                n350 = Select(t="Quece timeout", s=w833, f=w826) -> (s? t:f=w831:string)
                n351 = Format Into String(format string=": %s", initial string=w831, "mux10-1") -> (resulting string=w828:string)  [unwired: 1 in, 1 out]
                n352 = call "string log (SubVI).vi"("Enum"=enum16{"Init", "Log", "Read"}."Log", "state Name"=w828) -> ()  [unwired: 8 in, 2 out]
              }
              frame condition #1 {
              }
            }
            n353 = To Variant(anything="mux 10-1 data") -> (Variant=w821:variant)
            n354 = call "App enquece.vi"("command data"=w821, "command"="MEAS.mux10-1", "queue in"=w824) -> ("error out"=w818:errorcluster)  [unwired: 7 in, 1 out]
            n355 = Merge Errors(w819, w818) -> (w817:errorcluster)
          }
          event "request AC-all": Value Change {
            w840 = T8 {"eMIC 1"={"ACV"=0.0, "ACI"=0.0, "pF"=0.0, "kW"=0.0, "Freq"=0.0, "kvar"=0.0}, "eMIC 2"={"ACV"=0.0, "ACI"=0.0, "pF"=0.0, "kW"=0.0, "Freq"=0.0, "kvar"=0.0}, "eMIC 3"={"ACV"=0.0, "ACI"=0.0, "pF"=0.0, "kW"=0.0, "Freq"=0.0, "kvar"=0.0}, "eMIC 4"={"ACV"=0.0, "ACI"=0.0, "pF"=0.0, "kW"=0.0, "Freq"=0.0, "kvar"=0.0}, "eMIC 5"={"ACV"=0.0, "ACI"=0.0, "pF"=0.0, "kW"=0.0, "Freq"=0.0, "kvar"=0.0}, "eMIC 6"={"ACV"=0.0, "ACI"=0.0, "pF"=0.0, "kW"=0.0, "Freq"=0.0, "kvar"=0.0}}  # eMICs cluster
            n356 = event-data() -> ()  [unwired: 1 in, 1 out]
            n357 = disable-structure shown="LOGGING==TRUE" {
              disable-tunnel: w841 -> [w847 _]
              frame condition #0 (active) {
                n358 = Empty String/Path?(string/path=w847) -> (empty?=w854:bool)
                n359 = Select(t="Quece timeout", s=w854, f=w847) -> (s? t:f=w852:string)
                n360 = Format Into String(format string=": %s", initial string=w852, "request AC") -> (resulting string=w849:string)  [unwired: 1 in, 1 out]
                n361 = call "string log (SubVI).vi"("Enum"=enum16{"Init", "Log", "Read"}."Log", "state Name"=w849) -> ()  [unwired: 8 in, 2 out]
              }
              frame condition #1 {
              }
            }
            n362 = call "FGV wait for 6 eMICs.vi"("Enum"=enum16{"Init", "count"}."Init") -> ("error out"=w837:errorcluster)  [unwired: 8 in, 2 out]
            n363 = call "App enquece.vi"("error in (no error)"=w837, "command"="MEAS.requestAC", "queue in"=w846) -> ("error out"=w842:errorcluster)  [unwired: 7 in, 1 out]
            n364 = Merge Errors(w843, w842) -> (w839:errorcluster)
          }
          event User Event {
            n365 = event-data() -> ("Module ID"=w865:i32, "Array"=w880:T24[])  [unwired: 1 in]
            n366 = Variant To Data(type=0, Variant=w861) -> (data=w859:i32)  [unwired: 1 in, 1 out]
            n367 = for {
              tunnel: w880 -> [w943] mode=indexing
              shift-right: [w939] -> w856
              shift-left: T7 {"ACV"=0.0, "ACI"=0.0, "pF"=0.0, "kW"=0.0, "Freq"=0.0, "kvar"=0.0} ("eMIC response") -> [w941]
              n368 = Unbundle By Name(w943) -> ("float"=w940:dbl, "Name"=w942:string)
              n369 = case shown="\"kVar\"" w942 {
                tunnel: w941 -> [w944 w947 w950 w953 w956 w959 w962]
                tunnel: w940 -> [_ w945 w948 w951 w955 w957 w961]
                tunnel: [w944 w946 w949 w952 w954 w958 w960] -> w939
                frame "False", Default {
                }
                frame "ACI" {
                  n370 = Bundle By Name(cluster=w947, "ACI"=w945) -> (w946:T7)
                }
                frame "kW" {
                  n371 = Bundle By Name(cluster=w950, "kW"=w948) -> (w949:T7)
                }
                frame "PF" {
                  n372 = Bundle By Name(cluster=w953, "pF"=w951) -> (w952:T7)
                }
                frame "ACV" {
                  n373 = Bundle By Name(cluster=w956, "ACV"=w955) -> (w954:T7)
                }
                frame "Freq" {
                  n374 = Bundle By Name(cluster=w959, "Freq"=w957) -> (w958:T7)
                }
                frame "kVar" {
                  n375 = Bundle By Name(cluster=w962, "kvar"=w961) -> (w960:T7)
                }
              }
            }
            n376 = disable-structure shown="LOGGING==TRUE" {
              disable-tunnel: w866 -> [w917 _]
              disable-tunnel: w865 -> [w913 _]
              frame condition #0 (active) {
                n377 = Empty String/Path?(string/path=w917) -> (empty?=w919:bool)
                n378 = Select(t="Quece timeout", s=w919, f=w917) -> (s? t:f=w916:string)
                n379 = Format Into String(format string=":%s %d", initial string=w916, "CE14  data response", w913) -> (resulting string=w912:string)  [unwired: 1 in, 1 out]
                n380 = call "string log (SubVI).vi"("Enum"=enum16{"Init", "Log", "Read"}."Log", "state Name"=w912) -> ()  [unwired: 8 in, 2 out]
              }
              frame condition #1 {
              }
            }
            n381 = call "eMIC_calibration.vi"("eMIC data in"=w856) -> ("eMIC data out"=w855:T7)  [unwired: 10 in]
            n382 = case shown="6" w865 {
              tunnel: [w920 w922 w925 w928 w931 w934 w937] -> w871
              tunnel: w872 -> [w920 w923 w926 w929 w932 w935 w938]
              tunnel: w855 -> [_ w921 w924 w927 w930 w933 w936]
              frame 0, Default {
              }
              frame 1 {
                n383 = Bundle By Name(cluster=w923, "eMIC 1"=w921) -> (w922:T8)
              }
              frame 2 {
                n384 = Bundle By Name(cluster=w926, "eMIC 2"=w924) -> (w925:T8)
              }
              frame 3 {
                n385 = Bundle By Name(cluster=w929, "eMIC 3"=w927) -> (w928:T8)
              }
              frame 4 {
                n386 = Bundle By Name(cluster=w932, "eMIC 4"=w930) -> (w931:T8)
              }
              frame 5 {
                n387 = Bundle By Name(cluster=w935, "eMIC 5"=w933) -> (w934:T8)
              }
              frame 6 {
                n388 = Bundle By Name(cluster=w938, "eMIC 6"=w936) -> (w937:T8)
              }
            }
            n389 = case shown="1, Default" w859 {
              tunnel: w871 -> [w888 w906]
              tunnel: w870 -> [w887 _]
              tunnel: [w885 w904] -> w867
              tunnel: w863 -> [w884 w910]
              tunnel: [w883 w910] -> w862
              tunnel: w858 -> [w882 w907]
              tunnel: [w882 w907] -> w857
              frame 0 {
                n390 = call "FGV wait for 6 eMICs.vi"("Enum"=enum16{"Init", "count"}."count") -> ("error out"=w886:errorcluster, "wait done"=w889:bool)  [unwired: 8 in, 1 out]
                "AC  Completed" <- w889
                n391 = case shown="True" w889 {
                  tunnel: w888 -> [_ w899]
                  tunnel: w884 -> [w891 w897]
                  tunnel: w887 -> [w896 _]
                  tunnel: w886 -> [w893 w901]
                  tunnel: [w892 w900] -> w885
                  tunnel: [w891 w897] -> w883
                  frame False {
                    n392 = call "App enquece.vi"("Priority Enquece"=TRUE, "error in (no error)"=w893, "command"="Apps.WaitForEvent", "queue in"=w896) -> ("error out"=w892:errorcluster)  [unwired: 6 in, 1 out]
                  }
                  frame True {
                    n393 = To Variant(anything=w899) -> (Variant=w898:variant)
                    n394 = call "FGV Driver Data.vi"("DUT channel (1-11)"=w897, "Mode"=DUT_data_Mode."AC parameter", "error in (no error)"=w901, "FGV enum(Read)"=FGV_DRV_data."Write" ("FGV DRV data enum"), "data"=w898) -> ("error out"=w900:errorcluster)  [unwired: 3 in, 3 out]
                  }
                }
              }
              frame 1, Default {
                n395 = To Variant(anything=w906) -> (Variant=w905:variant)
                n396 = call "FGV Driver Data.vi"("Mode"=DUT_data_Mode."AC parameter 1", "DUT index(1-60)"=w907, "FGV enum(Read)"=FGV_DRV_data."Write", "data"=w905) -> ("error out"=w904:errorcluster)  [unwired: 4 in, 3 out]
              }
            }
            n397 = Unbundle By Name(w871) -> ("eMIC 1"=→"eMIC 1":T7, "eMIC 2"=→"eMIC 2":T7, "eMIC 3"=→"eMIC 3":T7, "eMIC 4"=→"eMIC 4":T7, "eMIC 5"=→"eMIC 5":T7, "eMIC 6"=→"eMIC 6":T7)
            n398 = Merge Errors(w868, w867) -> (w869:errorcluster)
          }
          event User Event {
            n399 = event-data() -> ("Init?"=w976:bool, "Module ID"=w963:i32)  [unwired: 1 in]
            "Module ID" <- w963
            "AC Measure Module" <- w976
            n400 = disable-structure shown="LOGGING==TRUE" {
              disable-tunnel: w978 -> [w998 _]
              disable-tunnel: w963 -> [w994 _]
              frame condition #0 (active) {
                n401 = Empty String/Path?(string/path=w998) -> (empty?=w1000:bool)
                n402 = Select(t="Quece timeout", s=w1000, f=w998) -> (s? t:f=w997:string)
                n403 = Format Into String(format string=":%s %d", initial string=w997, "CE14 Did  it", w994) -> (resulting string=w993:string)  [unwired: 1 in, 1 out]
                n404 = call "string log (SubVI).vi"("Enum"=enum16{"Init", "Log", "Read"}."Log", "state Name"=w993) -> ()  [unwired: 8 in, 2 out]
              }
              frame condition #1 {
              }
            }
            n405 = disable-structure shown="DEBUGGING==TRUE" {
              disable-tunnel: w963 -> [w1001 _]
              frame condition #0 {
                n406 = call "Show Panel.vi"("Module ID"=w1001) -> ()  [unwired: 10 in, 1 out]
              }
              frame condition #1 (active) {
              }
            }
            n407 = Decrement(x=w963) -> (x-1=w977:i32)
            n408 = Initialize Array(FALSE, 6 ("dimension size")) -> (w972:bool[])
            n409 = feedback #2(w972) -> (w973:bool[])
            n410 = Replace Array Subset(array=w973, new element=w976, index=w977) -> (w971:bool[])
            "CE14  Module did it" <- w971
            n411 = feedback-in #2(w971) -> ()
            n412 = And Array Elements(Boolean array=w971) -> (logical AND=w970:bool)
            n413 = case shown="False" w970 {
              tunnel: w969 -> [_ w985]
              tunnel: [_ w984] -> w968
              frame False {
              }
              frame True {
                n414 = flat-sequence {
                  tunnel: [w987] -> w986
                  tunnel: w985 -> [w987]
                  tunnel: w986 -> [w990]
                  tunnel: [w989] -> w984
                  frame #0 {
                    n415 = Wait (ms)(milliseconds to wait=u32 500) -> ()  [unwired: 1 out]
                  }
                  frame #1 {
                    n416 = call "App enquece.vi"("command"="MEAS.Read EMIC connected", "queue in"=w990) -> ("error out"=w989:errorcluster)  [unwired: 8 in, 1 out]
                  }
                }
              }
            }
            n417 = control-ref of="Select CE14 eMIC Module Instance"() -> (w983:refnum<vi>)
            n418 = call "Update Select Module Ring.vi"("Select Module Ring Ref"=w983) -> ("error out"=w967:errorcluster)  [unwired: 8 in, 2 out]
            n419 = Merge Errors(w979, w968, w967) -> (w980:errorcluster)
          }
          event "Shorted Circuits Test": Value Change {
            n420 = event-data() -> ()  [unwired: 1 in, 1 out]
            n421 = Build Array("Test Shorted Circuits") -> (w1007:string[])
            n422 = for {
              tunnel: [w1019] -> w1008 mode=indexing
              tunnel: w1007 -> [w1018] mode=indexing
              tunnel: w1006 -> [w1017]
              n423 = call "App enquece.vi"("command"=w1018, "queue in"=w1017) -> ("error out"=w1019:errorcluster)  [unwired: 8 in, 1 out]
            }
            n424 = Merge Errors(w1010, w1008) -> (w1009:errorcluster)
            n425 = disable-structure shown="Enabled" {
              frame Enabled {
                n426 = Initialize Array(FALSE, 6 ("dimension size"), 10 ("dimension size")) -> (w1013:bool[][])
                n427 = local write "Short DRV"(w1013) -> ()
              }
